vi "Main_09B.vi"() -> ()   [LabVIEW 2024]
panel:
  out "Count Down":i32
  out "Ending":cluster{"Array":i32[]}[](array[cluster])
  out "Starting":cluster{"Array":i32[]}[](array[cluster])
  out "original":cluster{"Array":i32[]}[](array[cluster])
  in  "Use Puzzle":bool
  out "Answer 6307279963620":u64
  in  "Puzzle":string="231044132293727419353356713211698585172072388022545729466698881739885330345853131193876427493925394014429761602571395381441257752012235131621368478541341764869712703015409959367852508018902266715148819874145969176460451991499162328927998859193886358553338987969221728049824729284712764041946274139389484987606762296286812070559741217532101358588036508666347111484425882317216983675862636276344366502048333862537413316779609175773596178350952698222837837476954334834078386840461362375326798489622437185066581969175658314639521022934457645459938617149663879828547848817873501493208119695668326092176931..."
  in  "Example":string="2333133121414131402"
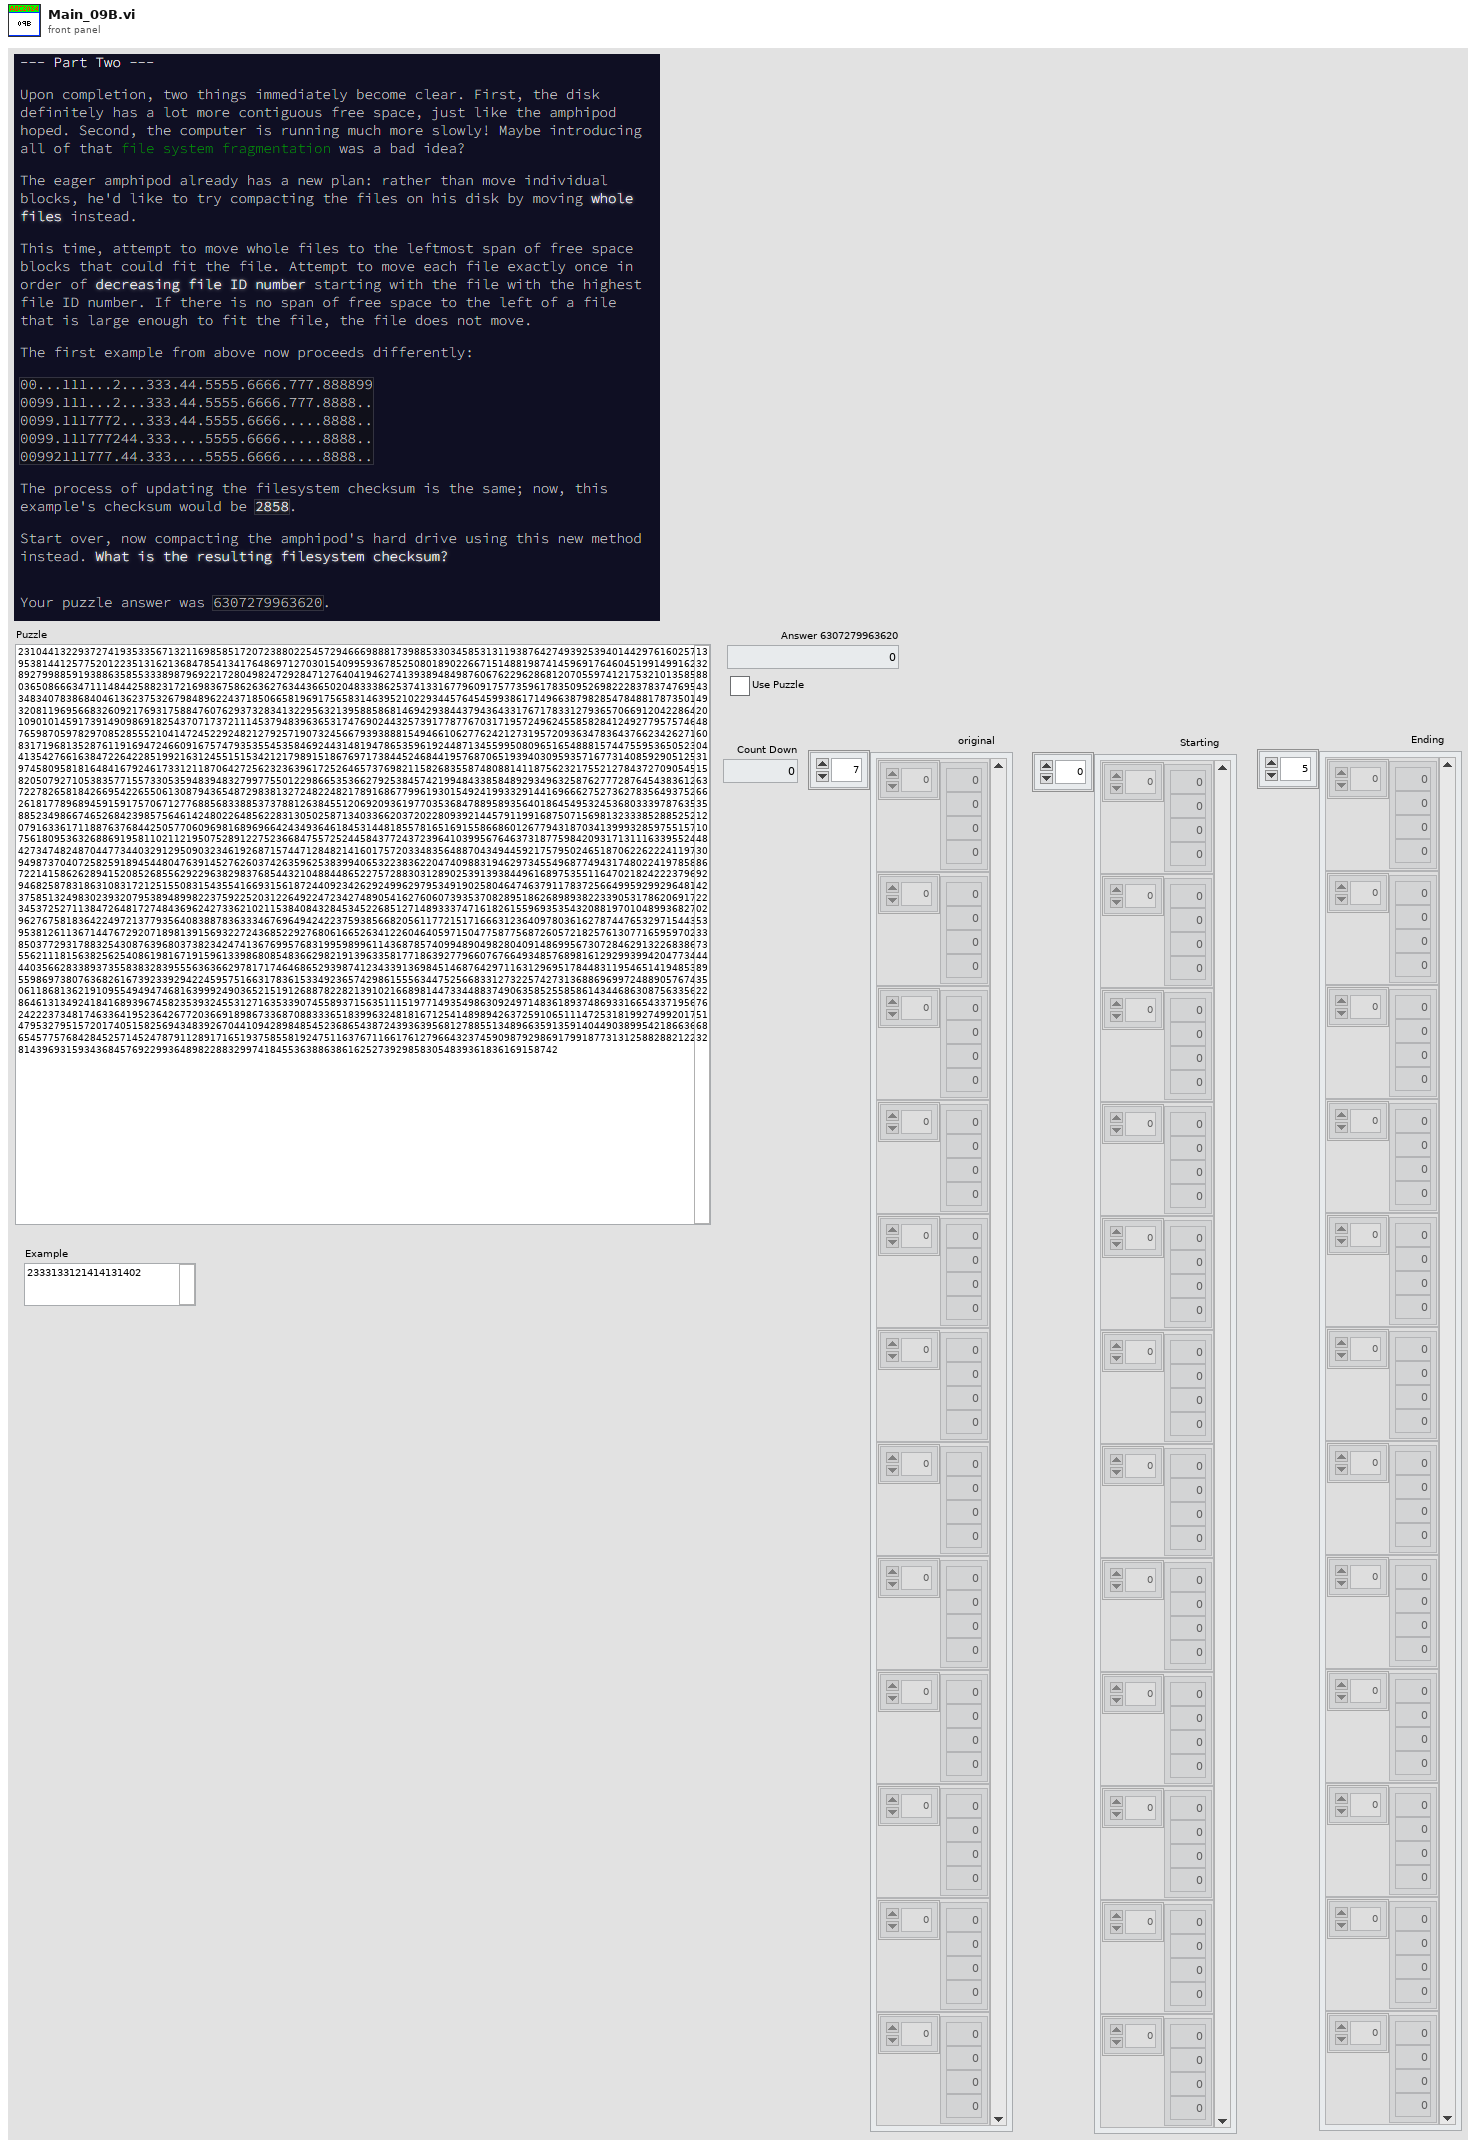
[diagram p1: front panel]
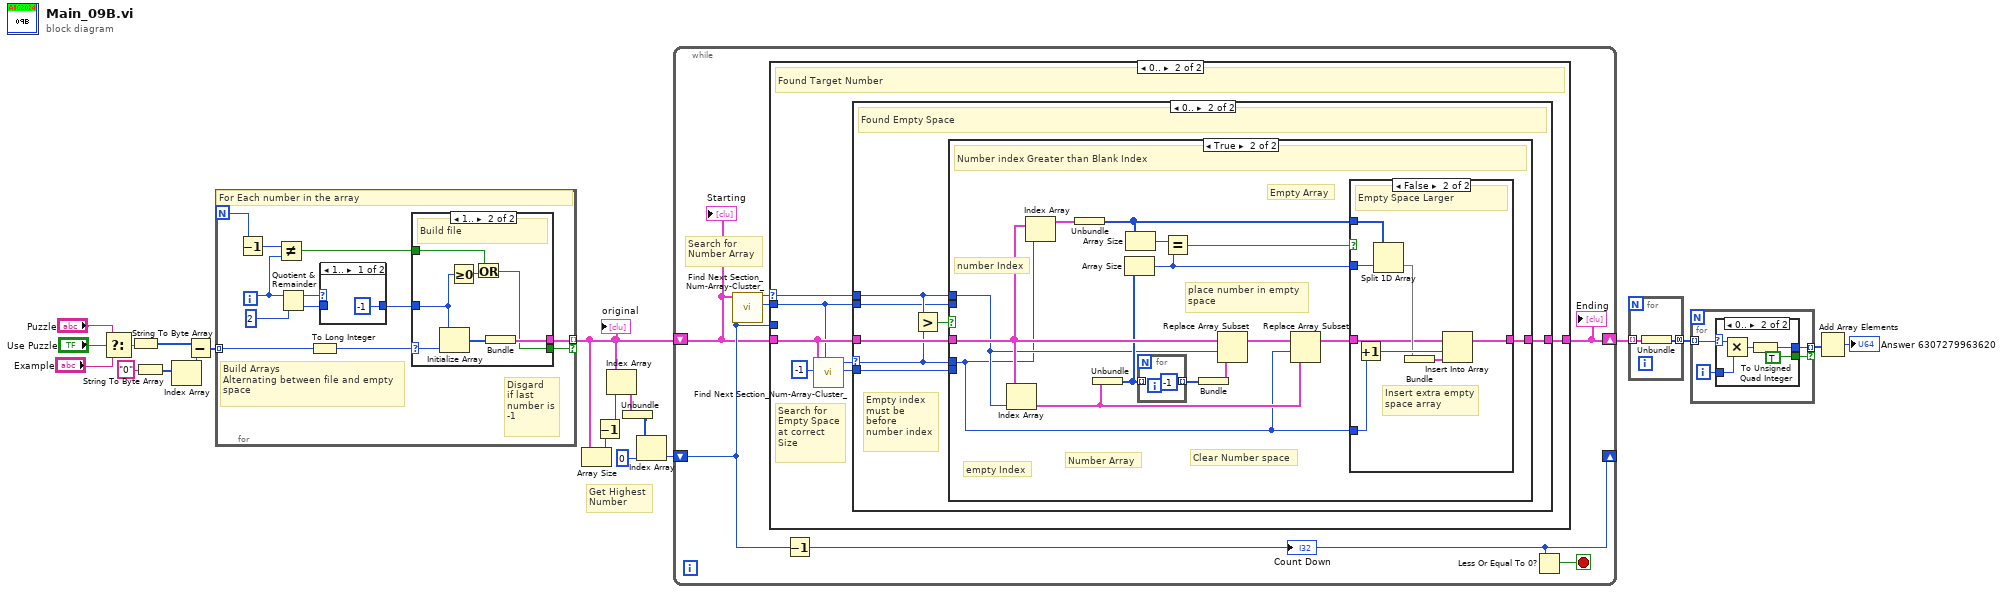
[diagram p0: block diagram]
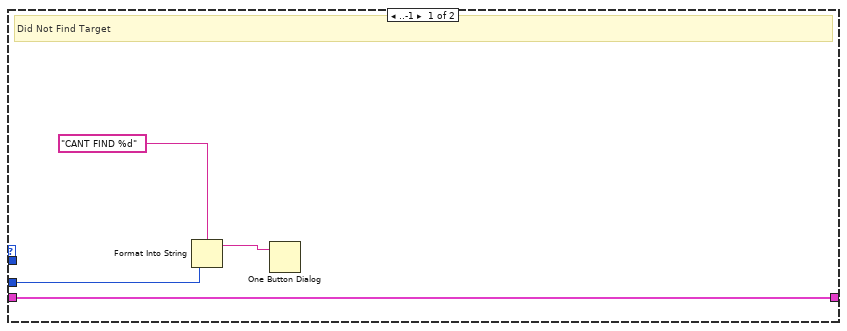
[diagram p2: hidden frame]
diagram:
  # "Get Highest\nNumber"
  n1 = Select(t="Puzzle", s="Use Puzzle", f="Example") -> (s? t:f=w16:string)
  n2 = String To Byte Array(string=w16) -> (unsigned byte array=w17:u8[])
  n3 = String To Byte Array(string="0") -> (unsigned byte array=w14:u8[])
  n4 = Index Array(array=w14) -> (element=w13:u8)  [unwired: 1 in]
  n5 = Subtract(x=w17, y=w13) -> (x-y=w12:u8[])
  n6 = for {
    N -> [w27]
    tunnel: w12 -> [w30] mode=indexing
    tunnel: [w22] -> w8 mode=indexing if=w21
    i -> [w25]
    # "Disgard\nif last\nnumber is\n-1"
    # "Build Arrays\nAlternating between file and empty\nspace"
    # "For Each number in the array"
    n7 = Decrement(x=w27) -> (x-1=w26:i32)
    n8 = Not Equal?(x=w26, y=w25) -> (x != y?=w24:bool)
    n9 = Quotient & Remainder(x=w25, y=2) -> (x-y*floor(x/y)=w31:i32, floor(x/y)=w29:i32)
    n10 = To Long Integer(number=w30) -> (32bit integer=w28:i32)
    n11 = case shown="1.." w31 {
      tunnel: w29 -> [_ w41]
      tunnel: [-1 w41] -> w23
      frame 1.. {
      }
      frame ..0 {
      }
    }
    n12 = case shown="1.." w28 {
      selector: w28 -> [_ w39]
      tunnel: w24 -> [_ w38]
      tunnel: w23 -> [_ w37]
      tunnel: [_ w34] -> w22
      tunnel: [_ w33] -> w21
      frame ..0 {
      }
      frame 1.. {
        # "Build file"
        n13 = Initialize Array(w37, w39) -> (w35:i32[])
        n14 = Greater Or Equal To 0?(x=w37) -> (x >= 0?=w36:bool)
        n15 = Or(x=w38, y=w36) -> (x .or. y?=w33:bool)
        n16 = Bundle(w35) -> (w34:cluster{i32[]})  [unwired: 1 in]
      }
    }
  }
  "original" <- w8
  n17 = Array Size(array=w8) -> (size(s)=w9:i32)
  n18 = Decrement(x=w9) -> (x-1=w7:i32)
  n19 = Index Array(array=w8, index=w7) -> (element=w6:cluster{i32[]})
  n20 = Unbundle(w6) -> (w5:i32[])
  n21 = Index Array(array=w5, index=0) -> (element=w3:i32)
  n22 = while {
    shift-right: [w42] -> w2
    shift-left: w8 -> [w43]
    shift-right: [w46] -> _
    shift-left: w3 -> [w44]
    stop <- w45 stop-if-true
    # "Search for\nNumber Array"
    n23 = call "Find Next Section_Num-Array-Cluster_.vi"("Find"=w44, "Array"=w43) -> ("Size Out"=w47:i32, "Index"=w48:i32)  [unwired: 7 in, 1 out]
    n24 = case shown="0.." w48 {
      selector: w48 -> [_ w58]
      tunnel: [w49 w59] -> w42
      tunnel: w43 -> [w49 w57]
      tunnel: w47 -> [_ w53]
      tunnel: w44 -> [w52 _]
      frame ..-1 {
        # "Did Not Find Target"
        n25 = Format Into String(format string="CANT FIND %d", w52) -> (resulting string=w50:string)  [unwired: 2 in, 1 out]
        n26 = One Button Dialog(message=w50) -> ()  [unwired: 1 in, 1 out]
      }
      frame 0.. {
        # "Search for\nEmpty Space\nat correct \nSize"
        # "Found Target Number"
        n27 = call "Find Next Section_Num-Array-Cluster_.vi"("Min Size"=w53, "Find"=-1 ("y"), "Array"=w57) -> ("Size Out"=w54:i32, "Index"=w55:i32)  [unwired: 6 in, 1 out]
        n28 = case shown="0.." w55 {
          selector: w55 -> [_ w64]
          tunnel: w58 -> [_ w65]
          tunnel: [w60 w67] -> w59
          tunnel: w57 -> [w60 w66]
          tunnel: w54 -> [_ w62]
          tunnel: w53 -> [_ w61]
          frame ..-1 {
            # "Did Not Find Empty Space"
          }
          frame 0.. {
            # "Empty index\nmust be \nbefore\nnumber index"
            # "Found Empty Space"
            n29 = Greater?(x=w65, y=w64) -> (0:w63:bool)
            n30 = case shown="True" w63 {
              tunnel: [w68 w78] -> w67
              tunnel: w66 -> [w68 w80]
              tunnel: w65 -> [_ w75]
              tunnel: w64 -> [_ w69]
              tunnel: w62 -> [_ _]
              tunnel: w61 -> [_ _]
              frame False {
                # "Blank Index is behind Number Index"
              }
              frame True {
                # "place number in empty\nspace"
                # "Number Array"
                # "Clear Number space"
                # "Empty Array"
                # "empty Index"
                # "number Index"
                # "Number index Greater than Blank Index"
                n31 = Index Array(array=w80, index=w75) -> (element=w70:cluster{i32[]})
                n32 = Index Array(array=w80, index=w69) -> (element=w83:cluster{i32[]})
                n33 = Unbundle(w83) -> (w73:i32[])
                n34 = Unbundle(w70) -> (w77:i32[])
                n35 = Array Size(array=w77) -> (size(s)=w74:i32)
                n36 = Array Size(array=w73) -> (size(s)=w76:i32)
                n37 = for {
                  tunnel: [-1] -> w81 mode=indexing
                  tunnel: w77 -> [_] mode=indexing
                }
                n38 = Equal?(x=w76, y=w74) -> (x = y?=w79:bool)
                n39 = Bundle(w81) -> (w82:cluster{i32[]})  [unwired: 1 in]
                n40 = Replace Array Subset(array=w80, new element=w82, index=w75) -> (w72:cluster{i32[]}[])
                n41 = Replace Array Subset(array=w72, new element=w70, index=w69) -> (w71:cluster{i32[]}[])
                n42 = case shown="False" w79 {
                  tunnel: w69 -> [_ w92]
                  tunnel: w73 -> [_ w89]
                  tunnel: w71 -> [w85 w86]
                  tunnel: [w85 w93] -> w78
                  tunnel: w74 -> [_ w90]
                  frame True {
                    # "Exact Fit"
                  }
                  frame False {
                    # "Insert extra empty\nspace array"
                    # "Empty Space Larger"
                    n43 = Increment(x=w92) -> (x+1=w91:i32)
                    n44 = Split 1D Array(array=w89, index=w90) -> (second subarray=w88:i32[])  [unwired: 1 out]
                    n45 = Bundle(w88) -> (w87:cluster{i32[]})  [unwired: 1 in]
                    n46 = Insert Into Array "Insert Into Array"(array=w86, index=w91, new element=w87) -> (w93:cluster{i32[]}[])
                  }
                }
              }
            }
          }
        }
      }
    }
    "Ending" <- w42
    n47 = Decrement(x=w44) -> (x-1=w46:i32)
    "Count Down" <- w46
    n48 = Less Or Equal To 0?(x=w46) -> (x <= 0?=w45:bool)
    "Starting" <- w43
  }
  n49 = for {
    tunnel: w2 -> [w95] mode=indexing
    tunnel: [w94] -> w1 mode=concatenating
    n50 = Unbundle(w95) -> (w94:i32[])
  }
  n51 = for {
    tunnel: w1 -> [w99] mode=indexing
    tunnel: [w97] -> w11 mode=indexing if=w96
    i -> [w98]
    n52 = case shown="0.." w99 {
      selector: w99 -> [_ w103]
      tunnel: w98 -> [_ w104]
      tunnel: [_ w100] -> w97
      tunnel: [_ TRUE] -> w96
      frame ..-1 {
      }
      frame 0.. {
        n53 = Multiply(x=w103, y=w104) -> (x*y=w102:i32)
        n54 = To Unsigned Quad Integer(1:w102) -> (0:w100:u64)
      }
    }
  }
  n55 = Add Array Elements(numeric array=w11) -> (sum=→"Answer 6307279963620":u64)
